vi "SetInitialBoard.vi"(8 "error in (no error)":errorcluster, 10 "InitialBoard":i32[][](array[numeric])=[[0, 0, 0, 0, 7, 0, 9, 4, 0], [0, 0, 0, 0, 9, 0, 0, 0, 5], [3, 0, 0, 0, 0, 5, 0, 7, 0], [0, 0, 7, 4, 0, 0, 1, 0, 0], [4, 6, 3, 0, 0, 0, 0, 0, 0], [0, 0, 0, 0, 0, 7, 0, 8, 0], [8, 0, 0, 0, 0, 0, 0, 0, 0], [7, 0, 0, 0, 0, 0, 0, 2, 8], [0, 5, 0, 2, 6, 0, 0, 0, 0]]) -> (0 "error out":errorcluster, 3 "SudukuBoard out":refnum<class "SudokuBoard.lvclass">)   [LabVIEW 2014, in "SudokuBoard.lvclass"]
uses:
  <userlib>/AdvancedDataStructures/ClassBased/Applications/SudukuSolver/SudukuBoard/SudokuBoard.lvclass
  <userlib>/AdvancedDataStructures/ClassBased/Applications/SudukuSolver/SudukuState/SudokuState.lvclass
  <userlib>/AdvancedDataStructures/ClassBased/Graph/Graph.lvclass
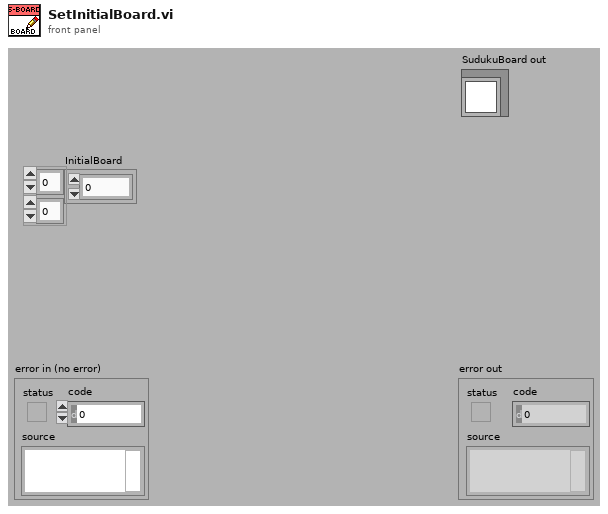
[diagram p1: front panel]
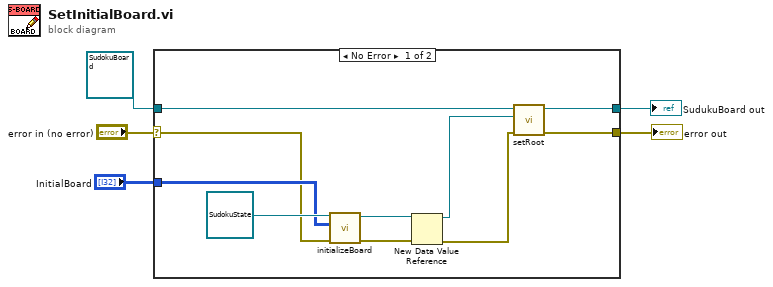
[diagram p0: block diagram]
diagram:
  n1 = case shown="No Error" "error in (no error)" {
    selector: "error in (no error)" -> [w9 w17]
    tunnel: [w6 w17] -> w4
    tunnel: [w10 w16] -> w2
    tunnel: refnum<class "SudokuBoard.lvclass"> refnum ("SudukuBoard in") -> [w11 w16]
    tunnel: "InitialBoard" -> [w12 _]
    frame No Error {
      n2 = call <userlib>:"initializeBoard.vi"("error in (no error)"=w9, "Board"=w12, "SudukuState in"=refnum<class "SudokuState.lvclass"> refnum ("SudukuState.lvclass")) -> ("error out"=w8:errorcluster, "SudukuState out"=w14:refnum<class "SudokuState.lvclass">)  [unwired: 7 in]
      n3 = New Data Value Reference(data value=w14, error in=w8) -> (data value reference=w13:refnum<data-value>, error out=w7:errorcluster)
      n4 = call <userlib>:"setRoot.vi"("error in (no error)"=w7, "Root"=w13, "Graph in"=w11) -> ("error out"=w6:errorcluster, "Graph out"=w10:refnum<class "SudokuBoard.lvclass">)  [unwired: 7 in]
    }
    frame Error {
    }
  }
  "error out" <- w4
  "SudukuBoard out" <- w2
